vi "WT_Single_Pass_analysis.vi"(2 "Radius":dbl=200.0, 3 "End Cut Deg":dbl, 4 "Start Cut Deg":dbl, 5 "Displacement":dbl[](array[numeric])) -> (0 "Blade Positions":dbl[](array[numeric]), 1 "Blade Angles":dbl[](array[numeric]))   [LabVIEW 2012]
uses:
  <vilib>/Analysis/baseanly.llb/Mean (DBL).vi
  <vilib>/Analysis/NI_AALPro.lvlib
  <vilib>/Analysis/NI_AALBase.lvlib
panel:
  out "Disp in":dbl[](graph)
  out "Blade 3":dbl[](graph)
  out "Blade 2":dbl[](graph)
  out "Blade1":dbl[](graph)
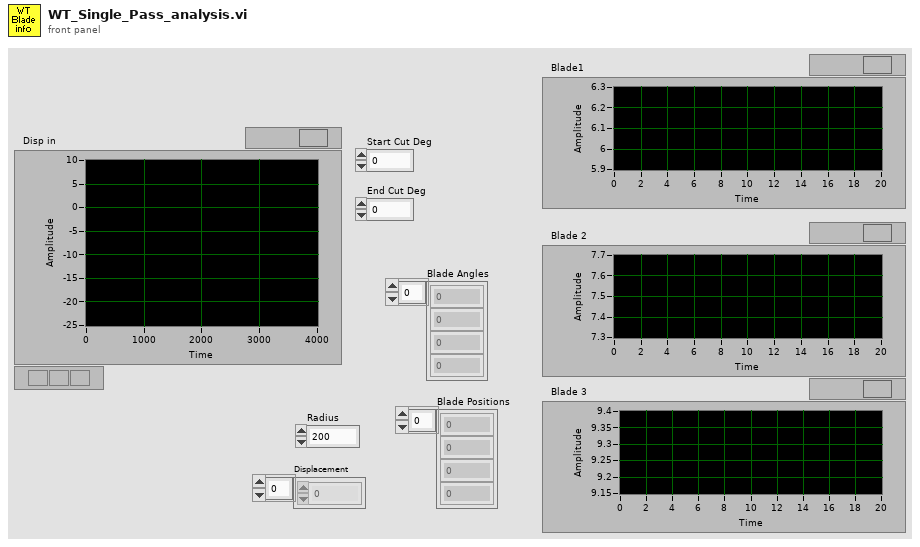
[diagram p1: front panel]
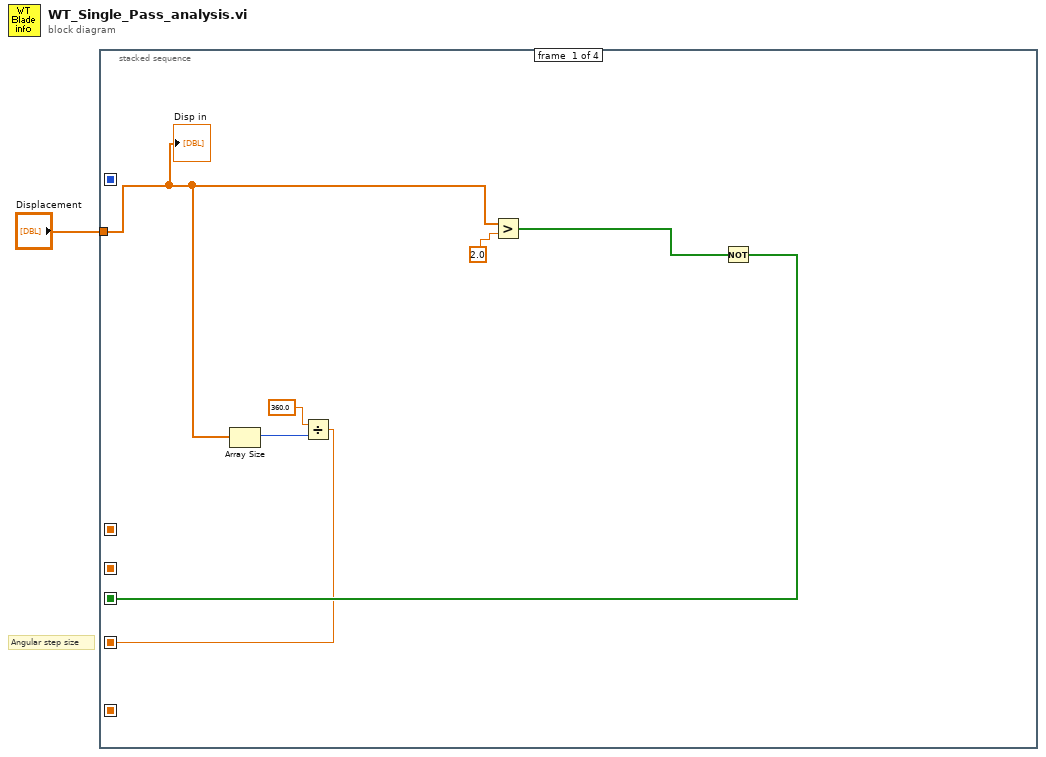
[diagram p0: block diagram]
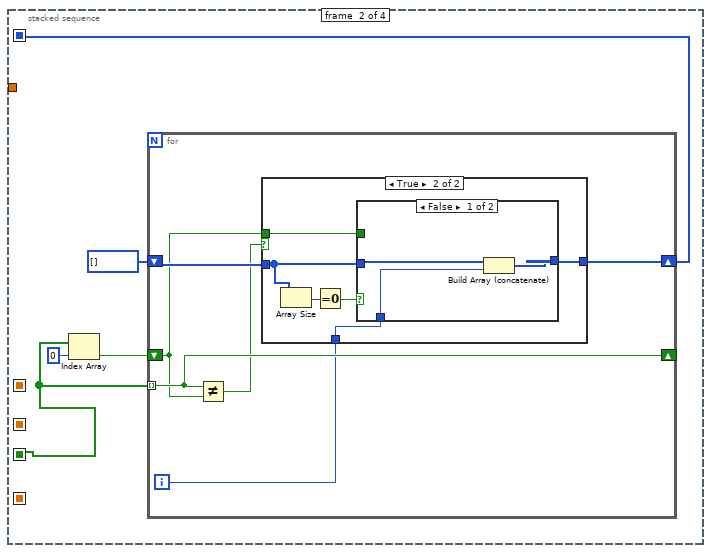
[diagram p2: hidden frame]
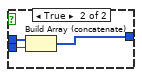
[diagram p5: hidden frame]
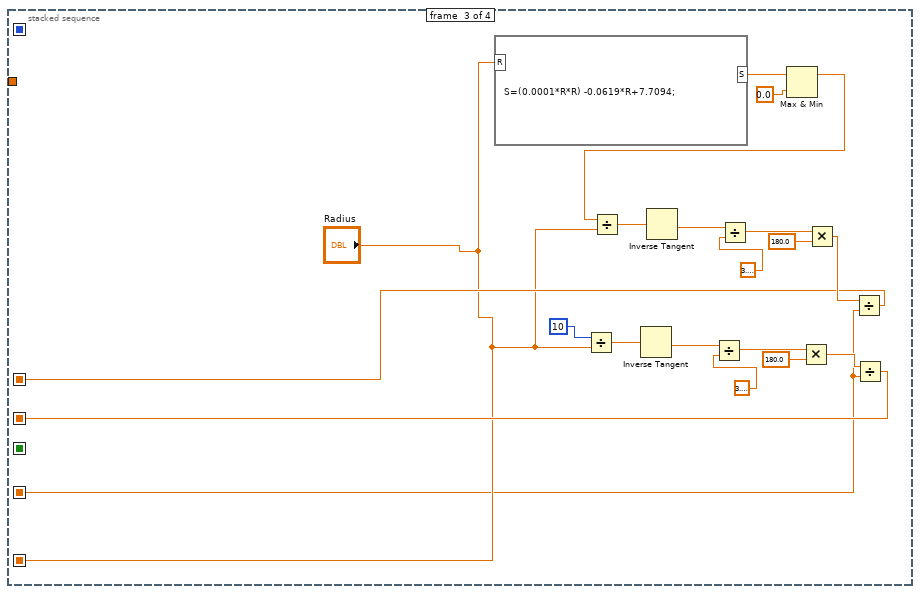
[diagram p6: hidden frame]
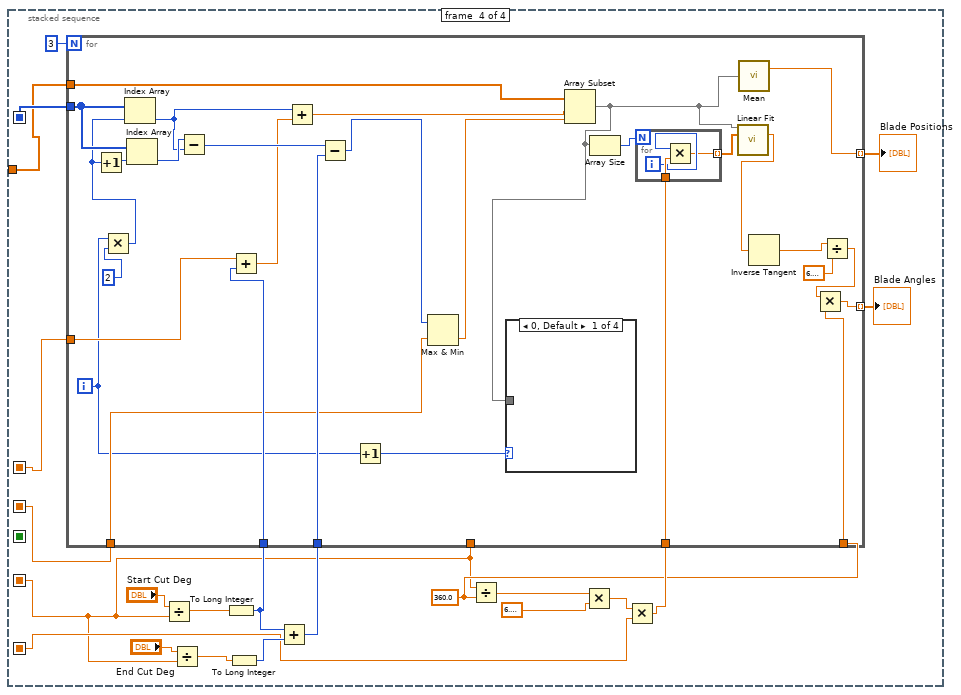
[diagram p7: hidden frame]
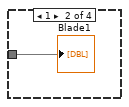
[diagram p8: hidden frame]
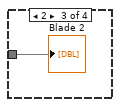
[diagram p9: hidden frame]
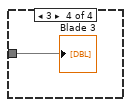
[diagram p10: hidden frame]
diagram:
  # "Angular step size"
  n1 = stacked-sequence {
    seq-local: [w8 _ _ _] -> [_ w9 _ _]
    seq-local: [_ w10 _ _] -> [_ _ _ w73]
    seq-local: [_ _ "Radius" _] -> [_ _ _ w64]
    seq-local: [_ _ w43 _] -> [_ _ _ w63]
    seq-local: [_ _ w45 _] -> [_ _ _ w62]
    seq-local: [w3 _ _ _] -> [_ _ w38 w58]
    tunnel: "Displacement" -> [w2 _ _ w61]
    frame #0 {
      n2 = Array Size(array=w2) -> (size(s)=w4:i32)
      n3 = Divide(x=360.0, y=w4) -> (x/y=w3:dbl)
      n4 = Greater?(x=w2, y=2.0) -> (0:w6:bool[])
      n5 = Not(x=w6) -> (.not. x?=w8:bool[])
      "Disp in" <- w2
    }
    frame #1 {
      n6 = Index Array(array=w9, index=0) -> (element=w12:bool)
      n7 = for {
        tunnel: w9 -> [w19] mode=indexing
        shift-right: [w19] -> _
        shift-left: w12 -> [w14]
        shift-right: [w16] -> w10
        shift-left: i32[] [] -> [w17]
        i -> [w18]
        n8 = Not Equal?(x=w19, y=w14) -> (x != y?=w15:bool)
        n9 = case shown="True" w15 {
          tunnel: w18 -> [_ w26]
          tunnel: w17 -> [w20 w24]
          tunnel: [w20 w25] -> w16
          tunnel: w14 -> [_ w21]
          frame False {
          }
          frame True {
            n10 = Array Size(array=w24) -> (size(s)=w23:i32)
            n11 = Equal To 0?(x=w23) -> (x = 0?=w22:bool)
            n12 = case shown="False" w22 {
              tunnel: w26 -> [w27 w33]
              tunnel: w24 -> [w29 w32]
              tunnel: [w28 w31] -> w25
              tunnel: w21 -> [_ w30]
              frame False {
                n13 = Build Array (concatenate)(w29, w27) -> (w28:i32[])
              }
              frame True {
                n14 = case shown="False" w30 {
                  tunnel: w33 -> [_ w37]
                  tunnel: w32 -> [w34 w36]
                  tunnel: [w34 w35] -> w31
                  frame False {
                  }
                  frame True {
                    n15 = Build Array (concatenate)(w36, w37) -> (w35:i32[])
                  }
                }
              }
            }
          }
        }
      }
    }
    frame #2 {
      n16 = formula code="S=(0.0001*R*R) -0.0619*R+7.7094;"("R"="Radius") -> ("S"=w42:dbl)
      n17 = Divide(x=10, y="Radius") -> (x/y=w56:dbl)
      n18 = Inverse Tangent(1:w56) -> (0:w55:dbl)
      n19 = Divide(x=w55, y=3.141592653589793) -> (x/y=w53:dbl)
      n20 = Max & Min(x=w42, y=0.0) -> (max(x,y)=w40:dbl)  [unwired: 1 out]
      n21 = Divide(x=w40, y="Radius") -> (x/y=w47:dbl)
      n22 = Inverse Tangent(1:w47) -> (0:w48:dbl)
      n23 = Divide(x=w48, y=3.141592653589793) -> (x/y=w50:dbl)
      n24 = Multiply(x=w53, y=180.0) -> (x*y=w44:dbl)
      n25 = Multiply(x=w50, y=180.0) -> (x*y=w46:dbl)
      n26 = Divide(x=w46, y=w38) -> (x/y=w45:dbl)
      n27 = Divide(x=w44, y=w38) -> (x/y=w43:dbl)
    }
    frame #3 {
      w65 = 360.0 ("y")
      n28 = Divide(x="Start Cut Deg", y=w58) -> (x/y=w75:dbl)
      n29 = Divide(x="End Cut Deg", y=w58) -> (x/y=w76:dbl)
      n30 = To Long Integer(number=w75) -> (32bit integer=w71:i32)
      n31 = To Long Integer(number=w76) -> (32bit integer=w74:i32)
      n32 = Add(x=w71, y=w74) -> (x+y=w70:i32)
      n33 = Divide(x=w58, y=w65) -> (x/y=w69:dbl)
      n34 = Multiply(x=w69, y=6.283185307179586) -> (x*y=w68:dbl)
      n35 = Multiply(x=w68, y=w64) -> (x*y=w66:dbl)
      n36 = for {
        N: 3 -> [_]
        tunnel: w61 -> [w104]
        tunnel: w73 -> [w101]
        tunnel: w71 -> [w90]
        tunnel: w70 -> [w97]
        tunnel: w66 -> [w96]
        tunnel: w65 -> [w91]
        tunnel: w58 -> [_]
        tunnel: w63 -> [w83]
        tunnel: w62 -> [w88]
        tunnel: [w86] -> w60 mode=indexing
        tunnel: [w85] -> w59 mode=indexing
        i -> [w81]
        n37 = Multiply(x=w81, y=2) -> (x*y=w99:i32)
        n38 = Increment(x=w99) -> (x+1=w98:i32)
        n39 = Index Array(array=w101, index=w99) -> (element=w106:i32)
        n40 = Index Array(array=w101, index=w98) -> (element=w107:i32)
        n41 = Subtract(x=w107, y=w106) -> (x-y=w105:i32)
        n42 = Add(x=w88, y=w90) -> (x+y=w89:dbl)
        n43 = Add(x=w106, y=w89) -> (x+y=w87:dbl)
        n44 = Subtract(x=w105, y=w97) -> (x-y=w84:i32)
        n45 = Increment(x=w81) -> (x+1=w79:i32)
        n46 = Max & Min(x=w84, y=w83) -> (min(x,y)=w82:dbl)  [unwired: 1 out]
        n47 = Array Subset(array=w104, index=w87, length=w82) -> (w80:dbl[])
        n48 = case shown="0, Default" w79 {
          tunnel: w80 -> [_ w108 w109 w110]
          frame 0, Default {
          }
          frame 1 {
            "Blade1" <- w108
          }
          frame 2 {
            "Blade 2" <- w109
          }
          frame 3 {
            "Blade 3" <- w110
          }
        }
        n49 = Array Size(array=w80) -> (size(s)=w103:i32)
        n50 = for {
          N: w103 -> [_]
          tunnel: w96 -> [w113]
          tunnel: [w111] -> w102 mode=indexing
          i -> [w112]
          n51 = Multiply(x=w112, y=w113) -> (x*y=w111:dbl)
        }
        n52 = call <vilib>:"Linear Fit.vi"("Y"=w80, "X"=w102) -> ("slope"=w95:dbl)  [unwired: 9 in, 4 out]
        n53 = call-poly <vilib>:"Mean.vi"("X"=w80) -> ("mean"=w85:dbl)  [unwired: 1 out]
        n54 = Inverse Tangent(1:w95) -> (0:w94:dbl)
        n55 = Divide(x=w94, y=6.283185307179586) -> (x/y=w92:dbl)
        n56 = Multiply(x=w92, y=w91) -> (x*y=w86:dbl)
      }
      "Blade Angles" <- w60
      "Blade Positions" <- w59
    }
  }
